vi "Check Instance Done.vi"(8 "error in (no error)":errorcluster, 11 "Log Instance in":T1) -> (0 "error out":errorcluster, 2 "Done?":bool, 3 "Log Instance out":T1)   [LabVIEW 2015, in "Waveform Log.lvclass"]
uses:
  Waveform Log.lvclass
  Log Instance.ctl
  Logs/Segmented Logs/Segmented Log/Segmented Log.lvclass
  Log Instance Waveform.ctl
  Waveform Information.ctl
  Waveform Data Type.ctl
  Logs/Segmented Logs/Segmented Log/Segmented Log.lvclass/Segmented Log.ctl
  Logs/Log Files/Log File/Log File.lvclass/Log File.ctl
  Logs/Log Files/TDMS Log File/TDMS Log File.lvclass/TDMS Log File.ctl
  Logs/Log Files/Text Log File/Text Log File.lvclass/Text Log File.ctl
  Logs/Segmented Logs/Segmented Log/Close Log File Instance.vi
  Logs/Log Files/Log File/Close Log File.vi
  Logs/Segmented Logs/Segmented Log/Make File Read-Only.vi
  Logs/Segmented Logs/Segmented Log/On Segmented Log Complete.vi
  Logs/Segmented Logs/Segmented Log/On File Close.vi
  Logs/Log Files/TDMS Log File/Close TDMS Log File.vi
  Logs/Log Files/Text Log File/Close Text Log File.vi
  Logs/Log Files/Log File/Log File.lvclass
  Logs/Log Files/TDMS Log File/TDMS Log File.lvclass
  Logs/Log Files/Text Log File/Text Log File.lvclass
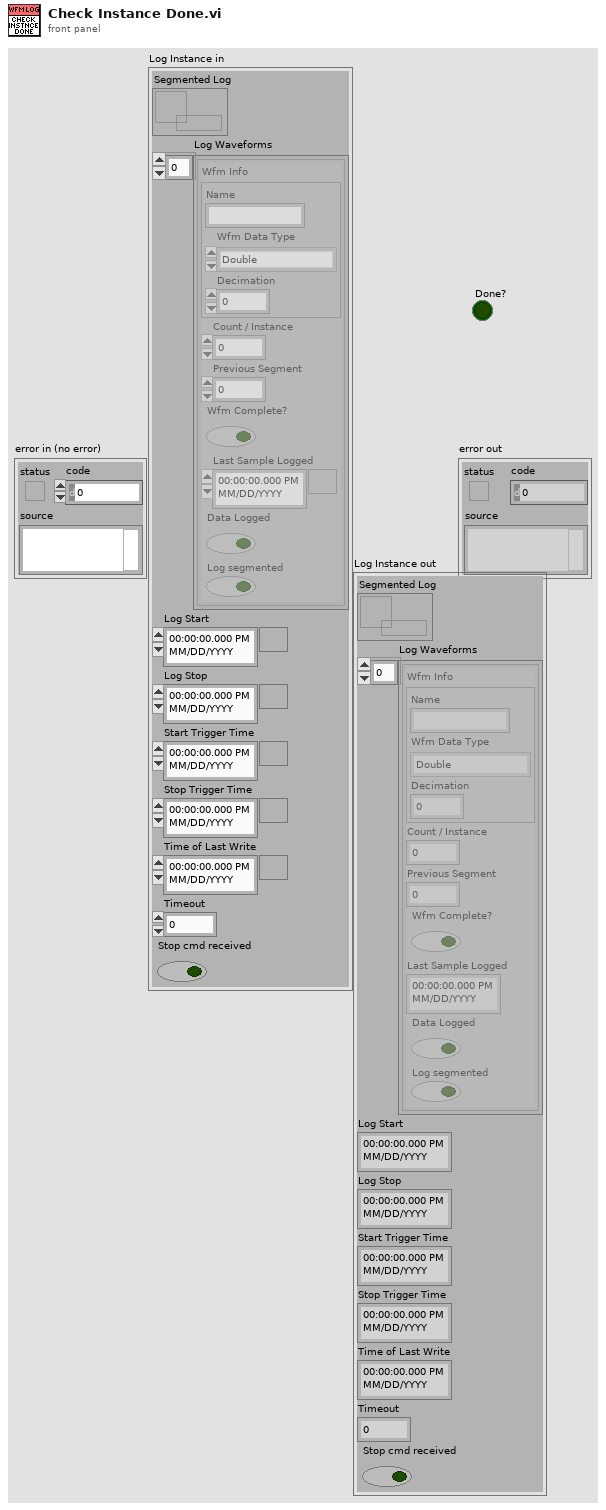
[diagram p1: front panel]
types:
  T1 = typedef "Waveform Log.lvclass/Log Instance.ctl" = cluster{"Segmented Log":refnum<data-value>, "Log Waveforms":T2[], "Log Start":timestamp, "Log Stop":timestamp, "Start Trigger Time":timestamp, "Stop Trigger Time":timestamp, "Time of Last Write":timestamp, "Timeout":dbl, "Stop cmd received":bool}
  T2 = typedef "Waveform Log.lvclass/Log Instance Waveform.ctl" = cluster{"Wfm Info":T3, "Count / Instance":i32, "Previous Segment":u64, "Wfm Complete?":bool, "Last Sample Logged":timestamp, "Data Logged":bool, "Log segmented":bool}
  T3 = typedef "Waveform Log.lvclass/Waveform Information.ctl" = cluster{"Name":string, "Wfm Data Type":T4, "Decimation":u32}
  T4 = typedef "Waveform Log.lvclass/Waveform Data Type.ctl" = enum16{"Double", "ComplexDouble"}
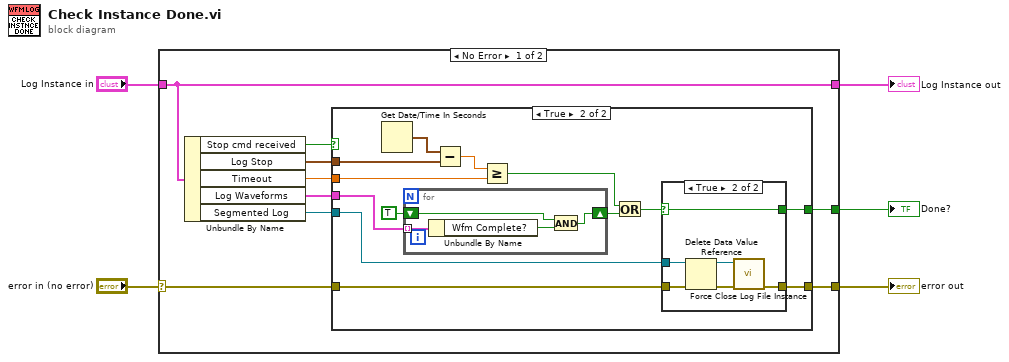
[diagram p0: block diagram]
diagram:
  n1 = case shown="No Error" "error in (no error)" {
    selector: "error in (no error)" -> [w12 w42]
    tunnel: [w11 w42] -> w4
    tunnel: "Log Instance in" -> [w8 w41]
    tunnel: [w9 _] -> w2
    tunnel: [w8 w41] -> w1
    frame No Error {
      n2 = Unbundle By Name(w8) -> ("Stop cmd received"=w6:bool, "Log Stop"=w7:timestamp, "Timeout"=w13:dbl, "Log Waveforms"=w14:T2[], "Segmented Log"=w10:refnum<data-value>)
      n3 = case shown="True" w6 {
        tunnel: w14 -> [_ w28]
        tunnel: w13 -> [_ w24]
        tunnel: w12 -> [w15 w23]
        tunnel: [w15 w22] -> w11
        tunnel: w10 -> [_ w21]
        tunnel: [_ w20] -> w9
        tunnel: w7 -> [_ w19]
        frame False {
        }
        frame True {
          n4 = Get Date/Time In Seconds() -> (seconds since 1Jan1904=w26:timestamp)
          n5 = for {
            tunnel: w28 -> [w40] mode=indexing
            shift-right: [w37] -> w17
            shift-left: TRUE -> [w38]
            n6 = Unbundle By Name(w40) -> ("Wfm Complete?"=w39:bool)
            n7 = And(x=w38, y=w39) -> (x .and. y?=w37:bool)
          }
          n8 = Subtract(x=w26, y=w19) -> (x-y=w25:dbl)
          n9 = Greater Or Equal?(x=w25, y=w24) -> (x >= y?=w18:bool)
          n10 = Or(x=w18, y=w17) -> (x .or. y?=w16:bool)
          n11 = case shown="True" w16 {
            selector: w16 -> [w30 w36]
            tunnel: w23 -> [w29 w35]
            tunnel: [w29 w31] -> w22
            tunnel: w21 -> [_ w33]
            tunnel: [w30 w36] -> w20
            frame False {
            }
            frame True {
              n12 = Delete Data Value Reference(data value reference=w33, error in=w35) -> (data value=w32:refnum<class "Segmented Log.lvclass">, error out=w34:errorcluster)
              n13 = call "Force Close Log File Instance.vi"("error in (no error)"=w34, "Segmented Log in"=w32) -> ("error out"=w31:errorcluster)  [unwired: 7 in, 2 out]
            }
          }
        }
      }
    }
    frame Error {
    }
  }
  "error out" <- w4
  "Done?" <- w2
  "Log Instance out" <- w1
